vi "Read Attributes.vi"(11 "File Data Msg":refnum<class "File Data Msg.lvclass">) -> (2 "Payload":cluster{"Data":string})   [LabVIEW 2018, in "Open File Actor.lvlib" / "File Data Msg.lvclass"]
uses:
  File Data Msg.lvclass
  File Data Msg.lvclass/File Data Msg.ctl
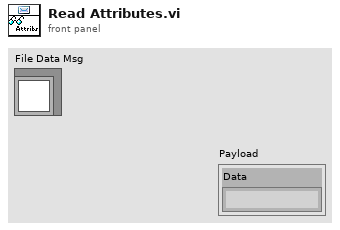
[diagram p1: front panel]
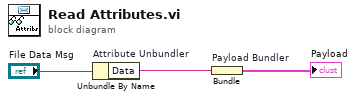
[diagram p0: block diagram]
diagram:
  n1 = Unbundle By Name "Attribute Unbundler"("File Data Msg") -> ("Data"=w1:string)
  n2 = Bundle "Payload Bundler"("Data"=w1) -> (→"Payload":cluster{"Data":string})  [unwired: 1 in]
